vi "WMP_test_CCL.vi"() -> ()   [LabVIEW 2013]
panel:
  out "status":string
  out "index":i32
  out "appended path":path
  out "filenames":string[](array[string])
  in  "Pause Button":bool
  in  "Vol.":i32(slide) min=0 max=100 step=1 scale=0.0..100.0
  in  "Skip Back Button":bool
  in  "Skip Forward Button":bool
  in  "Play Button":bool
  out "Number of Loop iterations":i32
  in  "stop":bool
  in  "currentPosition":dbl(slide) max=0.0 step=0.04 scale=0.0..1.0
  in  "WindowsMediaPlayer":refnum<k7>(container)
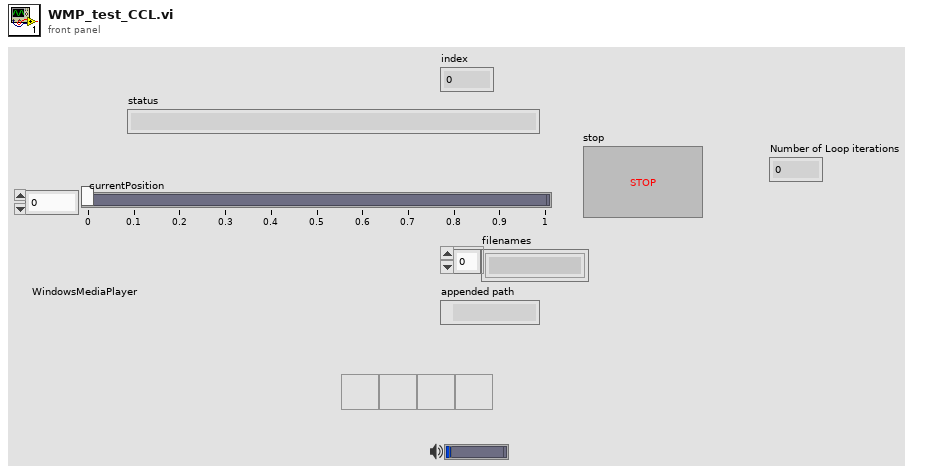
[diagram p1: front panel]
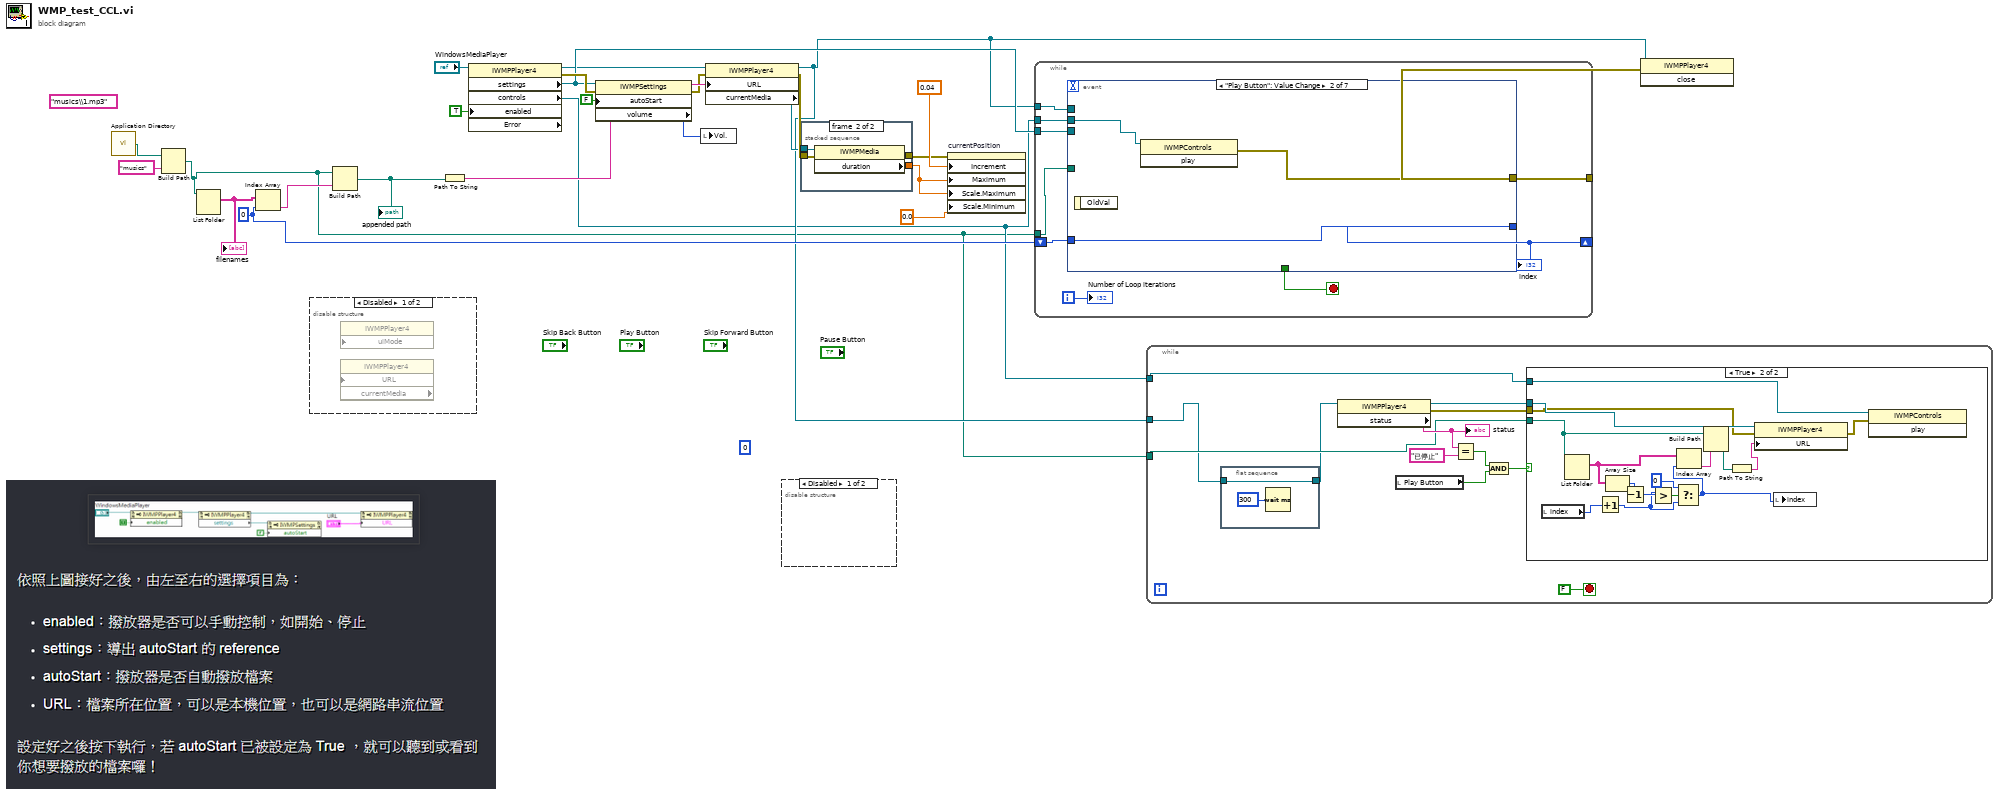
[diagram p0: block diagram]
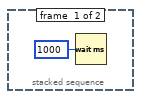
[diagram p5: hidden frame]
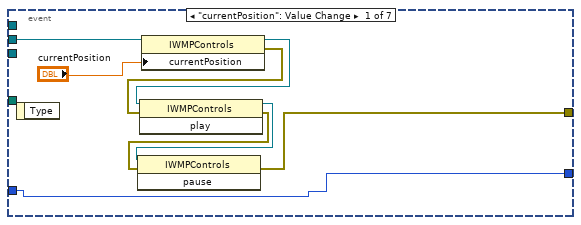
[diagram p6: hidden frame]
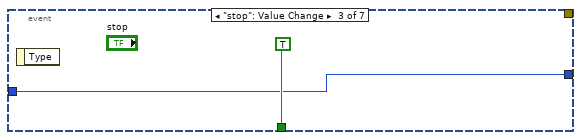
[diagram p7: hidden frame]
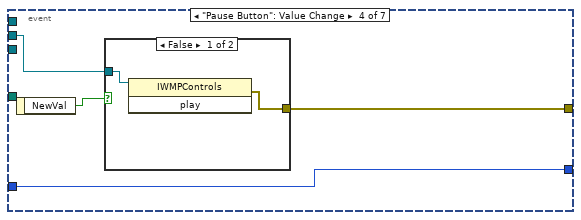
[diagram p8: hidden frame]
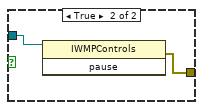
[diagram p9: hidden frame]
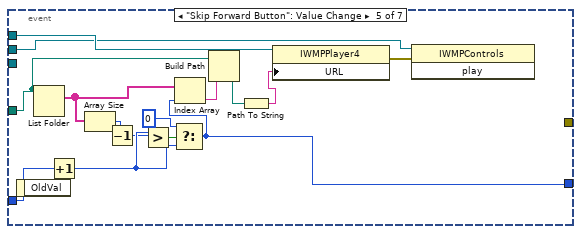
[diagram p10: hidden frame]
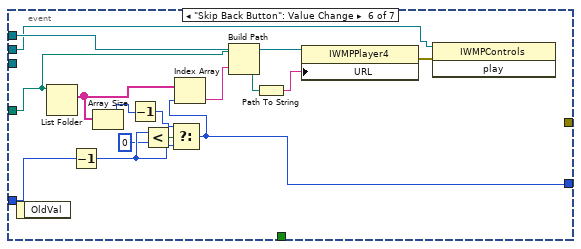
[diagram p11: hidden frame]
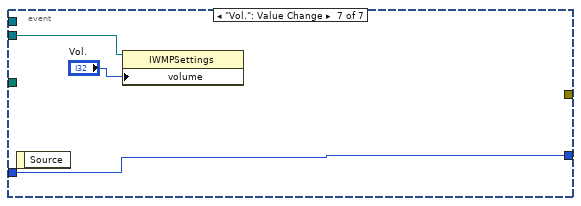
[diagram p12: hidden frame]
diagram:
  w4 = 0 ("index")
  (unwired) "musics\\1.mp3" ("name or relative path")
  (unwired) 0 ("volume")
  n1 = call <vilib>:"Application Directory.vi"() -> ("Application Directory"=w14:path)
  n2 = Build Path(base path=w14, name or relative path="musics") -> (appended path=w1:path)
  n3 = List Folder(path=w1) -> (filenames=w5:string[])  [unwired: 3 in, 3 out]
  "filenames" <- w5
  n4 = Index Array(array=w5, index=w4) -> (element=w6:string)
  n5 = disable-structure shown="Disabled" {
    frame Disabled {
      n6 = property class="IWMPPlayer4" props=["URL", "currentMedia"]() -> ()  [unwired: 3 in, 3 out]
      n7 = property class="IWMPPlayer4" props=["uiMode"]() -> ()  [unwired: 3 in, 2 out]
    }
    frame Enabled {
    }
  }
  n8 = Build Path(base path=w1, name or relative path=w6) -> (appended path=w7:path)
  "appended path" <- w7
  n9 = Path To String(path=w7) -> (string=w25:string)
  n10 = property class="IWMPPlayer4" props=["settings", "controls", "enabled", "Error"](reference="WindowsMediaPlayer", "enabled"=TRUE) -> (reference out=w8:refnum<k7>, error out=w18:errorcluster, "settings"=w12:refnum<k7>, "controls"=w2:refnum<k7>)  [unwired: 1 in, 1 out]
  n11 = property class="IWMPSettings"(reference=w12, error in=w18, "autoStart"=FALSE) -> (error out=w23:errorcluster, "volume"=w11:i32)  [unwired: 1 out]
  n12 = local write "Vol."(w11) -> ()
  n13 = property class="IWMPPlayer4"(reference=w8, error in=w23, "URL"=w25) -> (reference out=w3:refnum<k7>, error out=w16:errorcluster, "currentMedia"=w9:refnum<k7>)
  n14 = disable-structure shown="Disabled" {
    frame Disabled {
    }
    frame Enabled {
    }
  }
  n15 = stacked-sequence {
    tunnel: [_ w30] -> w21
    tunnel: [_ w29] -> w17
    tunnel: w16 -> [_ w28]
    tunnel: w9 -> [_ w27]
    frame #0 {
      n16 = Wait (ms)(milliseconds to wait=u32 1000) -> ()  [unwired: 1 out]
    }
    frame #1 {
      n17 = property class="IWMPMedia"(reference=w27, error in=w28) -> (error out=w29:errorcluster, "duration"=w30:dbl)  [unwired: 1 out]
    }
  }
  n18 = property on="currentPosition" class="Slide (strict)"(error in=w17, "Increment"=0.04 ("Data Entry Limits:Increment"), "Maximum"=w21, "Scale.Maximum"=w21, "Scale.Minimum"=0.0 ("Scale.Range:Minimum")) -> ()  [unwired: 1 in, 2 out]
  n19 = while {
    tunnel: w2 -> [w39]
    tunnel: [w38] -> w22
    tunnel: w12 -> [w35]
    shift-right: [w31] -> _
    shift-left: w4 -> [w34]
    tunnel: w1 -> [w33]
    tunnel: w3 -> [w32]
    i -> [w36]
    stop <- w37 stop-if-true
    n20 = event shown="[1] \"Play Button\": Value Change" {
      selector: _ -> [_ _ _ _ _ _ _]
      dyn-events: _ -> [_ _ _ _ _ _ _]
      timeout: _ -> [_ _ _ _ _ _ _]
      tunnel: w39 -> [w45 w50 _ w55 w62 w76 _]
      tunnel: [w43 w49 _ w54 _ _ _] -> w38
      tunnel: [_ _ TRUE _ _ _ _] -> w37
      tunnel: w35 -> [_ _ _ _ _ _ w92]
      tunnel: w34 -> [w40 w48 w51 w53 w74 w89 w91]
      tunnel: w33 -> [_ _ _ _ w68 w82 _]
      tunnel: w32 -> [_ _ _ _ w75 w90 _]
      tunnel: [w40 w48 w51 w53 w69 w84 w91] -> w31
      event "currentPosition": Value Change {
        n21 = event-data() -> ()  [unwired: 1 in, 1 out]
        n22 = property class="IWMPControls"(reference=w45, "currentPosition"="currentPosition") -> (reference out=w44:refnum<k7>, error out=w46:errorcluster)  [unwired: 1 in]
        n23 = invoke class="IWMPControls" method="play"(reference=w44, error in=w46) -> (reference out=w42:refnum<k7>, error out=w41:errorcluster)  [unwired: 1 in, 1 out]
        n24 = invoke class="IWMPControls" method="pause"(reference=w42, error in=w41) -> (error out=w43:errorcluster)  [unwired: 1 in, 2 out]
      }
      event "Play Button": Value Change {
        n25 = event-data() -> ()  [unwired: 1 in, 1 out]
        n26 = invoke class="IWMPControls" method="play"(reference=w50) -> (error out=w49:errorcluster)  [unwired: 2 in, 2 out]
      }
      event "stop": Value Change {
        n27 = event-data() -> ()  [unwired: 1 in, 1 out]
      }
      event "Pause Button": Value Change {
        n28 = event-data() -> ("NewVal"=w56:bool)  [unwired: 1 in]
        n29 = case shown="False" w56 {
          tunnel: w55 -> [w57 w60]
          tunnel: [w58 w59] -> w54
          frame False {
            n30 = invoke class="IWMPControls" method="play"(reference=w57) -> (error out=w58:errorcluster)  [unwired: 2 in, 2 out]
          }
          frame True {
            n31 = invoke class="IWMPControls" method="pause"(reference=w60) -> (error out=w59:errorcluster)  [unwired: 2 in, 2 out]
          }
        }
      }
      event "Skip Forward Button": Value Change {
        n32 = event-data() -> ()  [unwired: 1 in, 1 out]
        n33 = List Folder(path=w68) -> (filenames=w73:string[])  [unwired: 3 in, 3 out]
        n34 = Increment(x=w74) -> (x+1=w71:i32)
        n35 = Array Size(array=w73) -> (size(s)=w64:i32)
        n36 = Decrement(x=w64) -> (x-1=w63:i32)
        n37 = Greater?(x=w71, y=w63) -> (0:w72:bool)
        n38 = Select(t=0, s=w72, f=w71) -> (s? t:f=w69:i32)
        n39 = Index Array(array=w73, index=w69) -> (element=w67:string)
        n40 = Build Path(base path=w68, name or relative path=w67) -> (appended path=w66:path)
        n41 = Path To String(path=w66) -> (string=w65:string)
        n42 = property class="IWMPPlayer4"(reference=w75, "URL"=w65) -> (error out=w61:errorcluster)  [unwired: 1 in, 1 out]
        n43 = invoke class="IWMPControls" method="play"(reference=w62, error in=w61) -> ()  [unwired: 1 in, 3 out]
      }
      event "Skip Back Button": Value Change {
        n44 = event-data() -> ()  [unwired: 1 in, 1 out]
        n45 = List Folder(path=w82) -> (filenames=w88:string[])  [unwired: 3 in, 3 out]
        n46 = Decrement(x=w89) -> (x-1=w86:i32)
        n47 = Array Size(array=w88) -> (size(s)=w79:i32)
        n48 = Decrement(x=w79) -> (x-1=w78:i32)
        n49 = Less?(x=w86, y=0) -> (x < y?=w87:bool)
        n50 = Select(t=w78, s=w87, f=w86) -> (s? t:f=w84:i32)
        n51 = Index Array(array=w88, index=w84) -> (element=w80:string)
        n52 = Build Path(base path=w82, name or relative path=w80) -> (appended path=w83:path)
        n53 = Path To String(path=w83) -> (string=w81:string)
        n54 = property class="IWMPPlayer4"(reference=w90, "URL"=w81) -> (error out=w77:errorcluster)  [unwired: 1 in, 1 out]
        n55 = invoke class="IWMPControls" method="play"(reference=w76, error in=w77) -> ()  [unwired: 1 in, 3 out]
      }
      event "Vol.": Value Change {
        n56 = event-data() -> ()  [unwired: 1 in, 1 out]
        n57 = property class="IWMPSettings"(reference=w92, "volume"="Vol.") -> ()  [unwired: 1 in, 2 out]
      }
    }
    "index" <- w31
    "Number of Loop iterations" <- w36
  }
  n58 = while {
    tunnel: w3 -> [w95]
    tunnel: w2 -> [w100]
    tunnel: w1 -> [w97]
    stop <- FALSE stop-if-true
    n59 = flat-sequence {
      tunnel: w95 -> [w106]
      tunnel: [w106] -> w94
      frame #0 {
        n60 = Wait (ms)(milliseconds to wait=u32 300 ("millisecond multiple")) -> ()  [unwired: 1 out]
      }
    }
    n61 = property class="IWMPPlayer4"(reference=w94) -> (reference out=w98:refnum<k7>, error out=w96:errorcluster, "status"=w104:string)  [unwired: 1 in]
    "status" <- w104
    n62 = local read "Play Button"() -> (w101:bool)
    n63 = Equal?(x=w104, y="已停止") -> (x = y?=w102:bool)
    n64 = And(x=w102, y=w101) -> (x .and. y?=w99:bool)
    n65 = case shown="True" w99 {
      tunnel: w100 -> [_ w123]
      tunnel: w98 -> [_ w112]
      tunnel: w97 -> [_ w111]
      tunnel: w96 -> [_ w108]
      frame False {
      }
      frame True {
        n66 = local read "index"() -> (w114:i32)
        n67 = List Folder(path=w111) -> (filenames=w115:string[])  [unwired: 3 in, 3 out]
        n68 = Increment(x=w114) -> (x+1=w113:i32)
        n69 = Array Size(array=w115) -> (size(s)=w121:i32)
        n70 = Decrement(x=w121) -> (x-1=w122:i32)
        n71 = Greater?(x=w113, y=w122) -> (0:w116:bool)
        n72 = Select(t=0, s=w116, f=w113) -> (s? t:f=w109:i32)
        n73 = Index Array(array=w115, index=w109) -> (element=w118:string)
        n74 = Build Path(base path=w111, name or relative path=w118) -> (appended path=w119:path)
        n75 = Path To String(path=w119) -> (string=w120:string)
        n76 = property class="IWMPPlayer4"(reference=w112, error in=w108, "URL"=w120) -> (error out=w110:errorcluster)  [unwired: 1 out]
        n77 = local write "index"(w109) -> ()
        n78 = invoke class="IWMPControls" method="play"(reference=w123, error in=w110) -> ()  [unwired: 1 in, 3 out]
      }
    }
  }
  n79 = invoke class="IWMPPlayer4" method="close"(reference=w3, error in=w22) -> ()  [unwired: 1 in, 3 out]
